vi "Globals.vi"() -> ()   [LabVIEW 2011]
panel:
  out "EmerStop":bool
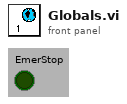
[diagram p1: front panel]
diagram:
